vi "List Mode - Read Configurations for Program Setup.vi"   [LabVIEW 2014, in "Associated Power Technologies 8500 Series.lvlib"]
uses:
  <instrlib>/Associated Power Technologies 8500 Series/Associated Power Technologies 8500 Series.lvlib
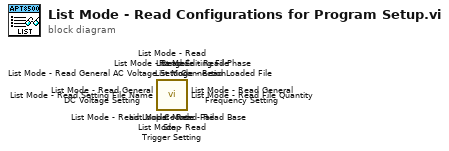
[diagram p0: block diagram]
diagram:
  n1 = call <instrlib>:"List Mode - Read Fail Stop.vi"() -> ()  [unwired: 9 in, 3 out]
  n2 = call <instrlib>:"List Mode - Read Phase Connection.vi"() -> ()  [unwired: 9 in, 3 out]
  n3 = call <instrlib>:"List Mode - Read General DC Voltage Setting.vi"() -> ()  [unwired: 9 in, 3 out]
  n4 = call <instrlib>:"List Mode - Read General Frequency Setting.vi"() -> ()  [unwired: 9 in, 3 out]
  n5 = call <instrlib>:"List Mode - Read General AC Voltage Setting.vi"() -> ()  [unwired: 9 in, 3 out]
  n6 = call <instrlib>:"List Mode - Read Range.vi"() -> ()  [unwired: 9 in, 3 out]
  n7 = call <instrlib>:"List Mode - Read Base.vi"() -> ()  [unwired: 9 in, 3 out]
  n8 = call <instrlib>:"List Mode - Read Trigger Setting.vi"() -> ()  [unwired: 9 in, 3 out]
  n9 = call <instrlib>:"List Mode - Read Loop Count.vi"() -> ()  [unwired: 9 in, 3 out]
  n10 = call <instrlib>:"List Mode - Read Setting File Name.vi"() -> ()  [unwired: 9 in, 3 out]
  n11 = call <instrlib>:"List Mode - Read File Quantity.vi"() -> ()  [unwired: 9 in, 3 out]
  n12 = call <instrlib>:"List Mode - Read Loaded File.vi"() -> ()  [unwired: 9 in, 3 out]
  n13 = call <instrlib>:"List Mode - Read Editing File.vi"() -> ()  [unwired: 9 in, 3 out]
